vi "FTW-Regex.vi"(0 "Regular Expression":string, 5 "Input String":string, 9 "Starting Offset":i32, 11 "error in":errorcluster) -> (4 "Match":string, 6 "Submatches":string[](array[string]), 8 "Match Found?":bool, 10 "Offset after Match":i32, 15 "error out":errorcluster)   [LabVIEW 2014]
uses:
  error/FTW-ERR-NoErrorConstant.vi
  error/FTW-ERR-CallChain.vi
  string/FTW-STR-ReplaceWhitespace.vi
  FTW-Regex.lvclass
panel:
  out "Match Offsets":i32[](array[numeric])
  # "Inputs"
  # "Debug"
  # "Outputs"
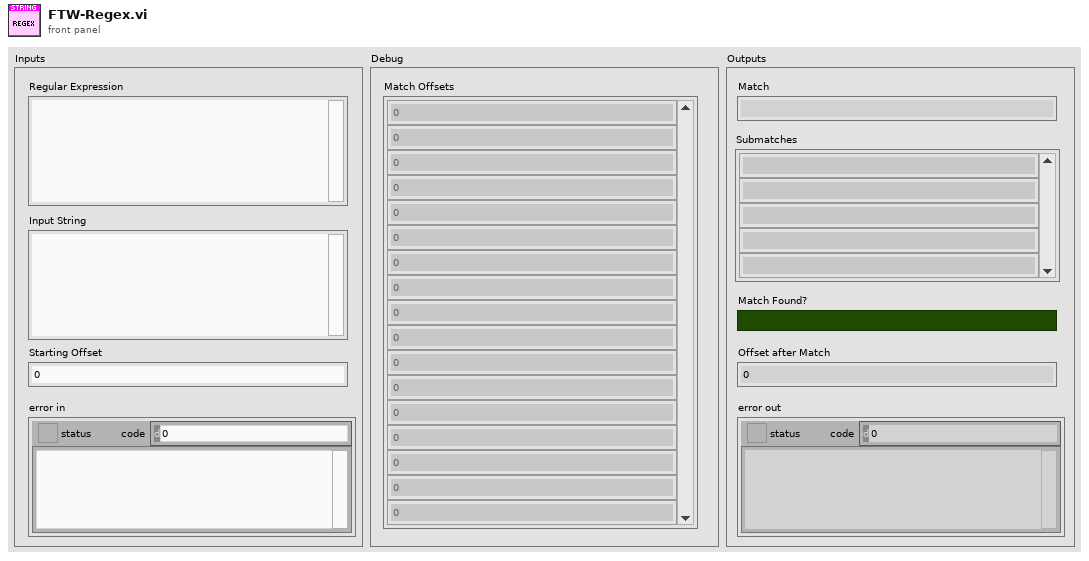
[diagram p1: front panel]
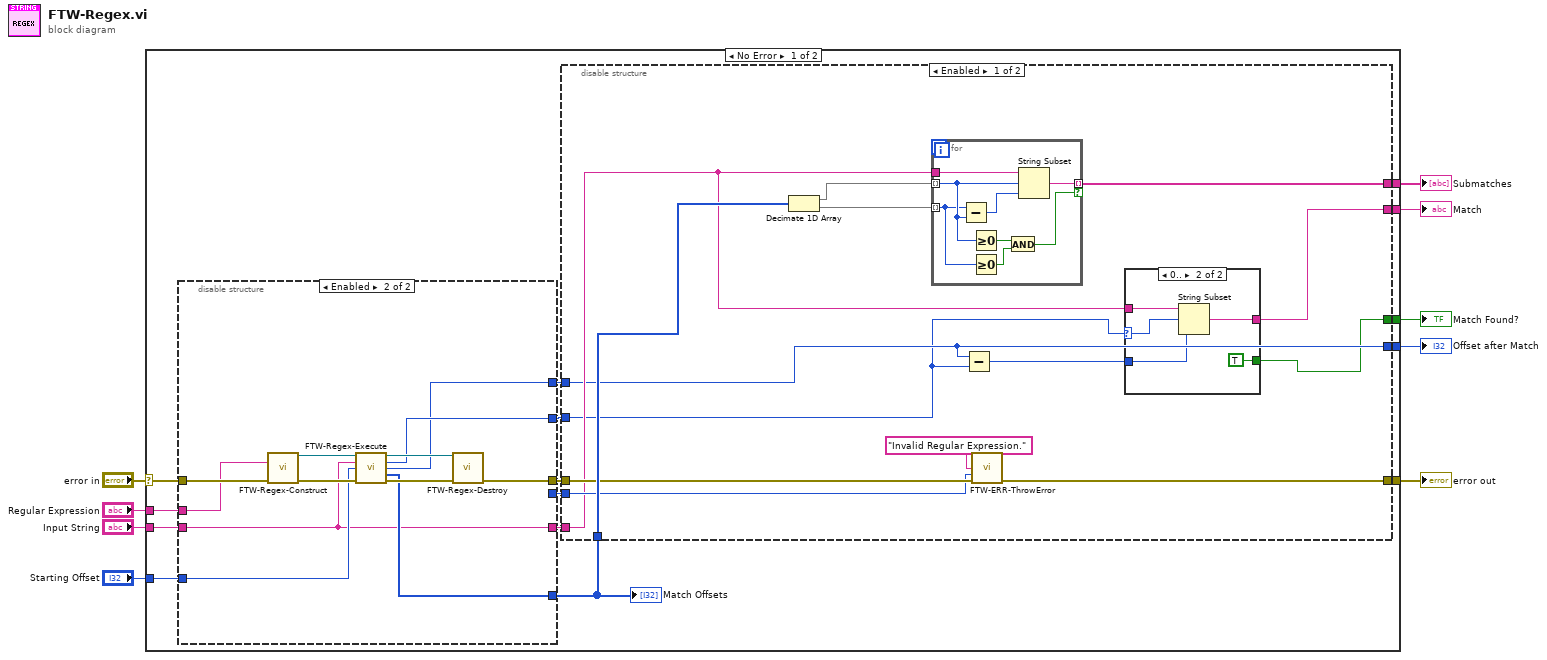
[diagram p0: block diagram]
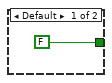
[diagram p2: hidden frame]
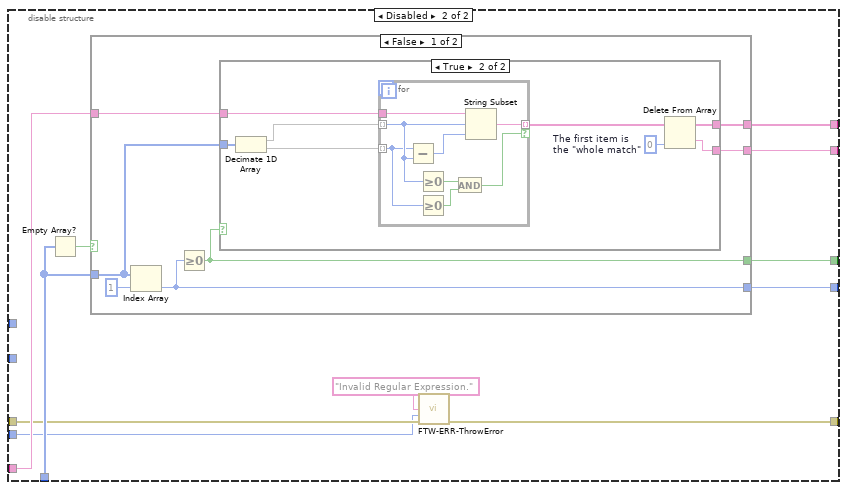
[diagram p3: hidden frame]
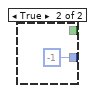
[diagram p5: hidden frame]
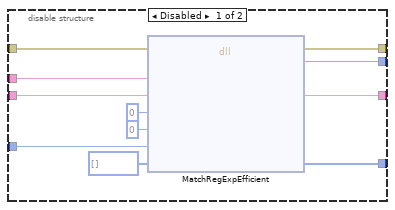
[diagram p6: hidden frame]
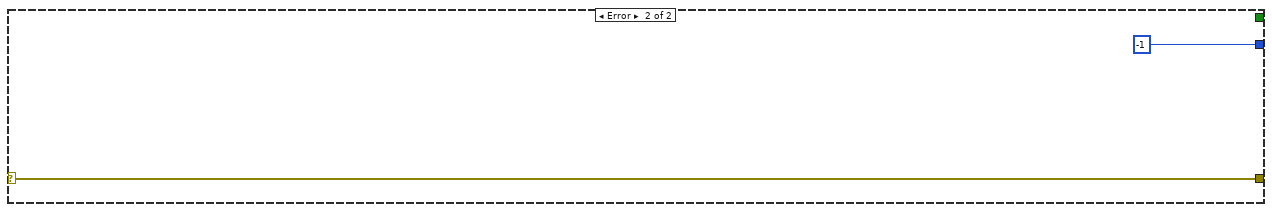
[diagram p7: hidden frame]
diagram:
  n1 = case shown="No Error" "error in" {
    selector: "error in" -> [w15 w111]
    tunnel: "Regular Expression" -> [w24 _]
    tunnel: [w23 _] -> w8
    tunnel: [w22 _] -> w7
    tunnel: [w13 w111] -> w6
    tunnel: "Starting Offset" -> [w21 _]
    tunnel: [w20 -1] -> w4
    tunnel: [w19 _] -> w3
    tunnel: "Input String" -> [w18 _]
    frame No Error {
      n2 = disable-structure shown="Enabled" {
        disable-tunnel: w24 -> [w98 w107]
        disable-tunnel: w21 -> [w97 w105]
        disable-tunnel: w18 -> [w96 w100]
        disable-tunnel: [w95 w100] -> w17
        disable-tunnel: [w91 w102] -> w16
        disable-tunnel: w15 -> [w90 w110]
        disable-tunnel: [w89 w106] -> w14
        disable-tunnel: [w88 _] -> w12
        disable-tunnel: [_ w101] -> w11
        disable-tunnel: [_ w99] -> w10
        frame Disabled {
          n3 = dll-call lib="LabVIEW" fn="MatchRegExpEfficient"(error in=w90, "Regular Expression"=w98, "Subject"=w96, "Ignore Case?"=0, "Multiline?"=0, "Starting Offset"=w97, "Match Offsets"=i32[] []) -> (error out=w89:errorcluster, "Return"=w88:i32, "Subject"=w95:string, "Match Offsets"=w91:i32[])  [unwired: 6 in, 1 out]
        }
        frame Enabled {
          n4 = call "FTW-Regex-Construct.vi"("Regular Expression"=w107, "error in"=w110) -> ("Regex"=w103:refnum<class "FTW-Regex.lvclass">, "error out"=w108:errorcluster)  [unwired: 12 in]
          n5 = call "FTW-Regex-Execute.vi"("Regex"=w103, "Subject String"=w100, "Starting Offset"=w105, "error in"=w108) -> ("Regex out"=w104:refnum<class "FTW-Regex.lvclass">, "Whole Match Begin"=w101:i32, "Offset after Match"=w99:i32, "Submatches"=w102:i32[], "error out"=w109:errorcluster)  [unwired: 6 in, 1 out]
          n6 = call "FTW-Regex-Destroy.vi"("Regex"=w104, "error in"=w109) -> ("error out"=w106:errorcluster)  [unwired: 13 in]
        }
      }
      "Match Offsets" <- w16
      n7 = disable-structure shown="Enabled" {
        disable-tunnel: [w29 w63] -> w23
        disable-tunnel: [w31 w62] -> w22
        disable-tunnel: [w28 w61] -> w20
        disable-tunnel: [w25 w60] -> w19
        disable-tunnel: w17 -> [w30 w59]
        disable-tunnel: w16 -> [w38 w58]
        disable-tunnel: w14 -> [w37 w56]
        disable-tunnel: [w36 w55] -> w13
        disable-tunnel: w12 -> [w35 w54]
        disable-tunnel: w11 -> [w26 _]
        disable-tunnel: w10 -> [w28 _]
        frame Enabled {
          n8 = Decimate 1D Array(w38) -> (w33:i32[], w32:i32[])
          n9 = for {
            tunnel: w30 -> [w52]
            tunnel: [w51] -> w31 mode=indexing if=w46
            tunnel: w33 -> [w49] mode=indexing
            tunnel: w32 -> [w45] mode=indexing
            n10 = Subtract(x=w45, y=w49) -> (x-y=w50:i32)
            n11 = Greater Or Equal To 0?(x=w49) -> (x >= 0?=w48:bool)
            n12 = Greater Or Equal To 0?(x=w45) -> (x >= 0?=w47:bool)
            n13 = And(x=w48, y=w47) -> (x .and. y?=w46:bool)
            n14 = String Subset(string=w52, offset (0)=w49, length (rest)=w50) -> (substring=w51:string)
          }
          n15 = Subtract(x=w28, y=w26) -> (x-y=w27:i32)
          n16 = call "FTW-ERR-ThrowError.vi"("Error Message"="Invalid Regular Expression.", "Error Code"=w35, "error in"=w37) -> ("error out"=w36:errorcluster)  [unwired: 12 in]
          n17 = case shown="0.." w26 {
            selector: w26 -> [_ w41]
            tunnel: w30 -> [_ w44]
            tunnel: [_ w43] -> w29
            tunnel: w27 -> [_ w42]
            tunnel: [FALSE TRUE] -> w25
            frame Default {
            }
            frame 0.. {
              n18 = String Subset(string=w44, offset (0)=w41, length (rest)=w42) -> (substring=w43:string)
            }
          }
        }
        frame Disabled {
          n19 = Empty Array?(array=w58) -> (empty?=w57:bool)
          n20 = case shown="False" w57 {
            tunnel: [w70 _] -> w63
            tunnel: [w69 _] -> w62
            tunnel: [w67 -1] -> w61
            tunnel: [w66 _] -> w60
            tunnel: w59 -> [w65 _]
            tunnel: w58 -> [w64 _]
            frame False {
              n21 = Index Array(array=w64, index=1) -> (element=w67:i32)
              n22 = Greater Or Equal To 0?(x=w67) -> (x >= 0?=w66:bool)
              n23 = case shown="True" w66 {
                tunnel: w65 -> [_ w78]
                tunnel: [_ w74] -> w70
                tunnel: [_ w73] -> w69
                tunnel: w64 -> [_ w71]
                frame False {
                }
                frame True {
                  w75 = 0  # The first item is the "whole match"
                  n24 = Decimate 1D Array(w71) -> (w77:i32[], w72:i32[])
                  n25 = for {
                    tunnel: w78 -> [w86]
                    tunnel: [w85] -> w76 mode=indexing if=w80
                    tunnel: w77 -> [w83] mode=indexing
                    tunnel: w72 -> [w79] mode=indexing
                    n26 = Subtract(x=w79, y=w83) -> (x-y=w84:i32)
                    n27 = Greater Or Equal To 0?(x=w83) -> (x >= 0?=w82:bool)
                    n28 = Greater Or Equal To 0?(x=w79) -> (x >= 0?=w81:bool)
                    n29 = And(x=w82, y=w81) -> (x .and. y?=w80:bool)
                    n30 = String Subset(string=w86, offset (0)=w83, length (rest)=w84) -> (substring=w85:string)
                  }
                  n31 = Delete From Array(array=w76, index=w75) -> (deleted portion=w74:string, array with subset deleted=w73:string[])  [unwired: 1 in]
                }
              }
            }
            frame True {
            }
          }
          n32 = call "FTW-ERR-ThrowError.vi"("Error Message"="Invalid Regular Expression.", "Error Code"=w54, "error in"=w56) -> ("error out"=w55:errorcluster)  [unwired: 12 in]
        }
      }
    }
    frame Error {
    }
  }
  "error out" <- w6
  "Submatches" <- w7
  "Match" <- w8
  "Match Found?" <- w3
  "Offset after Match" <- w4
